vi "Test at 5 second intervals.vi"() -> ()   [LabVIEW 2018]
uses:
  <vilib>/Plasmionique/MB Master/MB_Master_TCP/MB_Master_TCP.lvclass
  C:/Program Files (x86)/National Instruments/LabVIEW 2018/vi.lib/Plasmionique/MB Master/MB_Master/MB_Master.lvclass
  <vilib>/Plasmionique/MB Master/MB Master.lvlib
panel:
  in  "Delay Curtailment and Power Factor":bool
  in  "Stop Button":bool
  out "Done":bool
  in  "No Delay Curtailment and Power Factor":bool
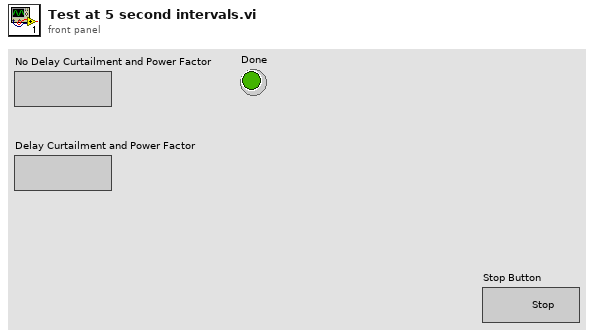
[diagram p1: front panel]
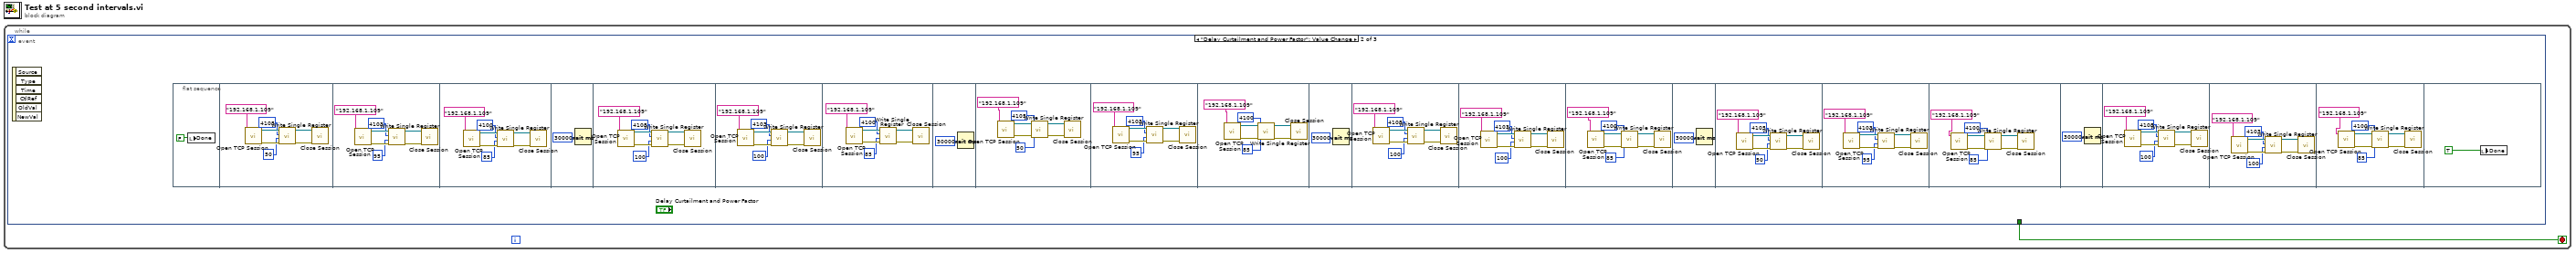
[diagram p0: block diagram]
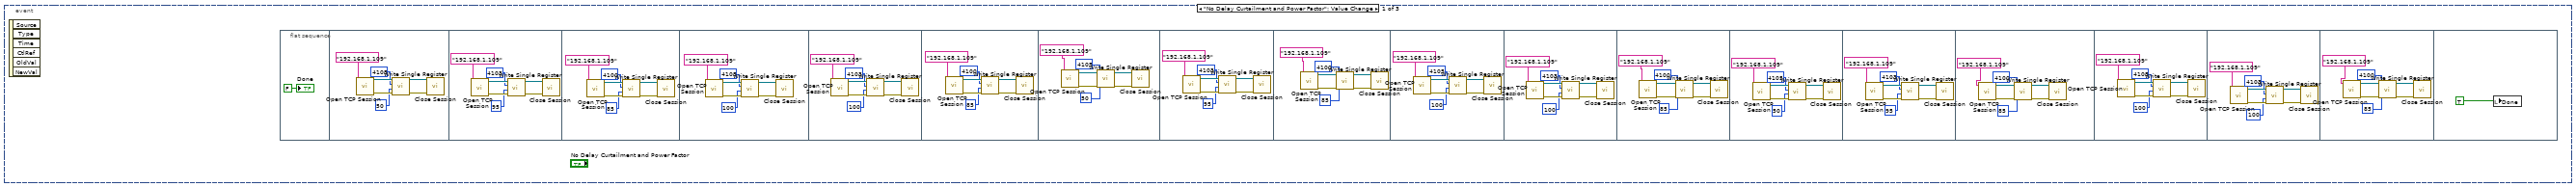
[diagram p2: hidden frame]
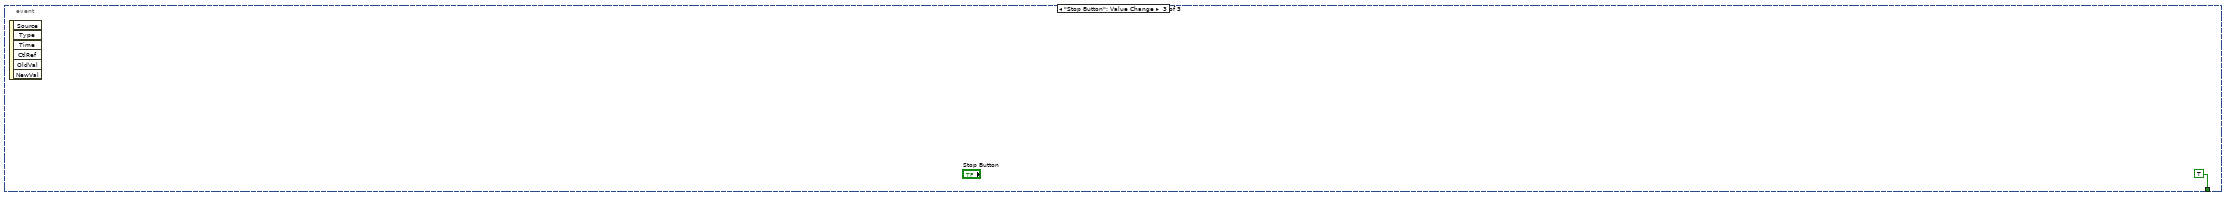
[diagram p3: hidden frame]
diagram:
  n1 = while {
    stop <- w1 stop-if-true
    n2 = event shown="[1] \"Delay Curtailment and Power Factor\": Value Change" {
      selector: _ -> [_ _ _]
      dyn-events: _ -> [_ _ _]
      timeout: _ -> [_ _ _]
      tunnel: [_ _ TRUE] -> w1
      event "No Delay Curtailment and Power Factor": Value Change {
        n3 = event-data() -> ()  [unwired: 1 in, 6 out]
        n4 = flat-sequence {
          frame #0 {
            "Done" <- FALSE ("Done")
          }
          frame #1 {
            n5 = call <vilib>:"Open TCP Session.vi"("IP Address"="192.168.1.109") -> ("error out"=w7:errorcluster, "MB_TCP session"=w9:refnum<class "MB_Master_TCP.lvclass">)  [unwired: 9 in]
            n6 = call <vilib>:"Write Single Register.vi"("error in (no error)"=w7, "value"=u16 50, "address"=u16 4105, "MB session in"=w9) -> ("error out"=w6:errorcluster, "MB session out"=w8:refnum<class "MB_Master_TCP.lvclass">)  [unwired: 6 in]
            n7 = call-dynamic "Close Session.vi"("error in (no error)"=w6, "MB TCP session"=w8) -> ()  [unwired: 9 in, 1 out]
          }
          frame #2 {
            n8 = call <vilib>:"Open TCP Session.vi"("IP Address"="192.168.1.109") -> ("error out"=w14:errorcluster, "MB_TCP session"=w16:refnum<class "MB_Master_TCP.lvclass">)  [unwired: 9 in]
            n9 = call <vilib>:"Write Single Register.vi"("error in (no error)"=w14, "value"=u16 95, "address"=u16 4103, "MB session in"=w16) -> ("error out"=w13:errorcluster, "MB session out"=w15:refnum<class "MB_Master_TCP.lvclass">)  [unwired: 6 in]
            n10 = call-dynamic "Close Session.vi"("error in (no error)"=w13, "MB TCP session"=w15) -> ()  [unwired: 9 in, 1 out]
          }
          frame #3 {
            n11 = call <vilib>:"Open TCP Session.vi"("IP Address"="192.168.1.109") -> ("error out"=w21:errorcluster, "MB_TCP session"=w23:refnum<class "MB_Master_TCP.lvclass">)  [unwired: 9 in]
            n12 = call <vilib>:"Write Single Register.vi"("error in (no error)"=w21, "value"=u16 85, "address"=u16 4100, "MB session in"=w23) -> ("error out"=w20:errorcluster, "MB session out"=w22:refnum<class "MB_Master_TCP.lvclass">)  [unwired: 6 in]
            n13 = call-dynamic "Close Session.vi"("error in (no error)"=w20, "MB TCP session"=w22) -> ()  [unwired: 9 in, 1 out]
          }
          frame #4 {
            n14 = call <vilib>:"Open TCP Session.vi"("IP Address"="192.168.1.109") -> ("error out"=w28:errorcluster, "MB_TCP session"=w30:refnum<class "MB_Master_TCP.lvclass">)  [unwired: 9 in]
            n15 = call <vilib>:"Write Single Register.vi"("error in (no error)"=w28, "value"=u16 100, "address"=u16 4105, "MB session in"=w30) -> ("error out"=w27:errorcluster, "MB session out"=w29:refnum<class "MB_Master_TCP.lvclass">)  [unwired: 6 in]
            n16 = call-dynamic "Close Session.vi"("error in (no error)"=w27, "MB TCP session"=w29) -> ()  [unwired: 9 in, 1 out]
          }
          frame #5 {
            n17 = call <vilib>:"Open TCP Session.vi"("IP Address"="192.168.1.109") -> ("error out"=w35:errorcluster, "MB_TCP session"=w37:refnum<class "MB_Master_TCP.lvclass">)  [unwired: 9 in]
            n18 = call <vilib>:"Write Single Register.vi"("error in (no error)"=w35, "value"=u16 100, "address"=u16 4103, "MB session in"=w37) -> ("error out"=w34:errorcluster, "MB session out"=w36:refnum<class "MB_Master_TCP.lvclass">)  [unwired: 6 in]
            n19 = call-dynamic "Close Session.vi"("error in (no error)"=w34, "MB TCP session"=w36) -> ()  [unwired: 9 in, 1 out]
          }
          frame #6 {
            n20 = call <vilib>:"Open TCP Session.vi"("IP Address"="192.168.1.109") -> ("error out"=w42:errorcluster, "MB_TCP session"=w44:refnum<class "MB_Master_TCP.lvclass">)  [unwired: 9 in]
            n21 = call <vilib>:"Write Single Register.vi"("error in (no error)"=w42, "value"=u16 85, "address"=u16 4100, "MB session in"=w44) -> ("error out"=w41:errorcluster, "MB session out"=w43:refnum<class "MB_Master_TCP.lvclass">)  [unwired: 6 in]
            n22 = call-dynamic "Close Session.vi"("error in (no error)"=w41, "MB TCP session"=w43) -> ()  [unwired: 9 in, 1 out]
          }
          frame #7 {
            n23 = call <vilib>:"Open TCP Session.vi"("IP Address"="192.168.1.109") -> ("error out"=w50:errorcluster, "MB_TCP session"=w48:refnum<class "MB_Master_TCP.lvclass">)  [unwired: 9 in]
            n24 = call <vilib>:"Write Single Register.vi"("error in (no error)"=w50, "value"=u16 50, "address"=u16 4105, "MB session in"=w48) -> ("error out"=w51:errorcluster, "MB session out"=w49:refnum<class "MB_Master_TCP.lvclass">)  [unwired: 6 in]
            n25 = call-dynamic "Close Session.vi"("error in (no error)"=w51, "MB TCP session"=w49) -> ()  [unwired: 9 in, 1 out]
          }
          frame #8 {
            n26 = call <vilib>:"Open TCP Session.vi"("IP Address"="192.168.1.109") -> ("error out"=w56:errorcluster, "MB_TCP session"=w58:refnum<class "MB_Master_TCP.lvclass">)  [unwired: 9 in]
            n27 = call <vilib>:"Write Single Register.vi"("error in (no error)"=w56, "value"=u16 95, "address"=u16 4103, "MB session in"=w58) -> ("error out"=w55:errorcluster, "MB session out"=w57:refnum<class "MB_Master_TCP.lvclass">)  [unwired: 6 in]
            n28 = call-dynamic "Close Session.vi"("error in (no error)"=w55, "MB TCP session"=w57) -> ()  [unwired: 9 in, 1 out]
          }
          frame #9 {
            n29 = call <vilib>:"Open TCP Session.vi"("IP Address"="192.168.1.109") -> ("error out"=w63:errorcluster, "MB_TCP session"=w65:refnum<class "MB_Master_TCP.lvclass">)  [unwired: 9 in]
            n30 = call <vilib>:"Write Single Register.vi"("error in (no error)"=w63, "value"=u16 85, "address"=u16 4100, "MB session in"=w65) -> ("error out"=w62:errorcluster, "MB session out"=w64:refnum<class "MB_Master_TCP.lvclass">)  [unwired: 6 in]
            n31 = call-dynamic "Close Session.vi"("error in (no error)"=w62, "MB TCP session"=w64) -> ()  [unwired: 9 in, 1 out]
          }
          frame #10 {
            n32 = call <vilib>:"Open TCP Session.vi"("IP Address"="192.168.1.109") -> ("error out"=w70:errorcluster, "MB_TCP session"=w72:refnum<class "MB_Master_TCP.lvclass">)  [unwired: 9 in]
            n33 = call <vilib>:"Write Single Register.vi"("error in (no error)"=w70, "value"=u16 100, "address"=u16 4105, "MB session in"=w72) -> ("error out"=w69:errorcluster, "MB session out"=w71:refnum<class "MB_Master_TCP.lvclass">)  [unwired: 6 in]
            n34 = call-dynamic "Close Session.vi"("error in (no error)"=w69, "MB TCP session"=w71) -> ()  [unwired: 9 in, 1 out]
          }
          frame #11 {
            n35 = call <vilib>:"Open TCP Session.vi"("IP Address"="192.168.1.109") -> ("error out"=w77:errorcluster, "MB_TCP session"=w79:refnum<class "MB_Master_TCP.lvclass">)  [unwired: 9 in]
            n36 = call <vilib>:"Write Single Register.vi"("error in (no error)"=w77, "value"=u16 100, "address"=u16 4103, "MB session in"=w79) -> ("error out"=w76:errorcluster, "MB session out"=w78:refnum<class "MB_Master_TCP.lvclass">)  [unwired: 6 in]
            n37 = call-dynamic "Close Session.vi"("error in (no error)"=w76, "MB TCP session"=w78) -> ()  [unwired: 9 in, 1 out]
          }
          frame #12 {
            n38 = call <vilib>:"Open TCP Session.vi"("IP Address"="192.168.1.109") -> ("error out"=w84:errorcluster, "MB_TCP session"=w86:refnum<class "MB_Master_TCP.lvclass">)  [unwired: 9 in]
            n39 = call <vilib>:"Write Single Register.vi"("error in (no error)"=w84, "value"=u16 85, "address"=u16 4100, "MB session in"=w86) -> ("error out"=w83:errorcluster, "MB session out"=w85:refnum<class "MB_Master_TCP.lvclass">)  [unwired: 6 in]
            n40 = call-dynamic "Close Session.vi"("error in (no error)"=w83, "MB TCP session"=w85) -> ()  [unwired: 9 in, 1 out]
          }
          frame #13 {
            n41 = call <vilib>:"Open TCP Session.vi"("IP Address"="192.168.1.109") -> ("error out"=w91:errorcluster, "MB_TCP session"=w93:refnum<class "MB_Master_TCP.lvclass">)  [unwired: 9 in]
            n42 = call <vilib>:"Write Single Register.vi"("error in (no error)"=w91, "value"=u16 50, "address"=u16 4105, "MB session in"=w93) -> ("error out"=w90:errorcluster, "MB session out"=w92:refnum<class "MB_Master_TCP.lvclass">)  [unwired: 6 in]
            n43 = call-dynamic "Close Session.vi"("error in (no error)"=w90, "MB TCP session"=w92) -> ()  [unwired: 9 in, 1 out]
          }
          frame #14 {
            n44 = call <vilib>:"Open TCP Session.vi"("IP Address"="192.168.1.109") -> ("error out"=w98:errorcluster, "MB_TCP session"=w100:refnum<class "MB_Master_TCP.lvclass">)  [unwired: 9 in]
            n45 = call <vilib>:"Write Single Register.vi"("error in (no error)"=w98, "value"=u16 95, "address"=u16 4103, "MB session in"=w100) -> ("error out"=w97:errorcluster, "MB session out"=w99:refnum<class "MB_Master_TCP.lvclass">)  [unwired: 6 in]
            n46 = call-dynamic "Close Session.vi"("error in (no error)"=w97, "MB TCP session"=w99) -> ()  [unwired: 9 in, 1 out]
          }
          frame #15 {
            n47 = call <vilib>:"Open TCP Session.vi"("IP Address"="192.168.1.109") -> ("error out"=w105:errorcluster, "MB_TCP session"=w107:refnum<class "MB_Master_TCP.lvclass">)  [unwired: 9 in]
            n48 = call <vilib>:"Write Single Register.vi"("error in (no error)"=w105, "value"=u16 85, "address"=u16 4100, "MB session in"=w107) -> ("error out"=w104:errorcluster, "MB session out"=w106:refnum<class "MB_Master_TCP.lvclass">)  [unwired: 6 in]
            n49 = call-dynamic "Close Session.vi"("error in (no error)"=w104, "MB TCP session"=w106) -> ()  [unwired: 9 in, 1 out]
          }
          frame #16 {
            n50 = call <vilib>:"Open TCP Session.vi"("IP Address"="192.168.1.109") -> ("error out"=w112:errorcluster, "MB_TCP session"=w114:refnum<class "MB_Master_TCP.lvclass">)  [unwired: 9 in]
            n51 = call <vilib>:"Write Single Register.vi"("error in (no error)"=w112, "value"=u16 100, "address"=u16 4105, "MB session in"=w114) -> ("error out"=w111:errorcluster, "MB session out"=w113:refnum<class "MB_Master_TCP.lvclass">)  [unwired: 6 in]
            n52 = call-dynamic "Close Session.vi"("error in (no error)"=w111, "MB TCP session"=w113) -> ()  [unwired: 9 in, 1 out]
          }
          frame #17 {
            n53 = call <vilib>:"Open TCP Session.vi"("IP Address"="192.168.1.109") -> ("error out"=w119:errorcluster, "MB_TCP session"=w121:refnum<class "MB_Master_TCP.lvclass">)  [unwired: 9 in]
            n54 = call <vilib>:"Write Single Register.vi"("error in (no error)"=w119, "value"=u16 100, "address"=u16 4103, "MB session in"=w121) -> ("error out"=w118:errorcluster, "MB session out"=w120:refnum<class "MB_Master_TCP.lvclass">)  [unwired: 6 in]
            n55 = call-dynamic "Close Session.vi"("error in (no error)"=w118, "MB TCP session"=w120) -> ()  [unwired: 9 in, 1 out]
          }
          frame #18 {
            n56 = call <vilib>:"Open TCP Session.vi"("IP Address"="192.168.1.109") -> ("error out"=w126:errorcluster, "MB_TCP session"=w128:refnum<class "MB_Master_TCP.lvclass">)  [unwired: 9 in]
            n57 = call <vilib>:"Write Single Register.vi"("error in (no error)"=w126, "value"=u16 85, "address"=u16 4100, "MB session in"=w128) -> ("error out"=w125:errorcluster, "MB session out"=w127:refnum<class "MB_Master_TCP.lvclass">)  [unwired: 6 in]
            n58 = call-dynamic "Close Session.vi"("error in (no error)"=w125, "MB TCP session"=w127) -> ()  [unwired: 9 in, 1 out]
          }
          frame #19 {
            n59 = local write "Done"(TRUE ("No Delay Curtailment")) -> ()
          }
        }
      }
      event "Delay Curtailment and Power Factor": Value Change {
        n60 = event-data() -> ()  [unwired: 1 in, 6 out]
        n61 = flat-sequence {
          frame #0 {
            n62 = local write "Done"(FALSE ("Done")) -> ()
          }
          frame #1 {
            n63 = call <vilib>:"Open TCP Session.vi"("IP Address"="192.168.1.109") -> ("error out"=w135:errorcluster, "MB_TCP session"=w137:refnum<class "MB_Master_TCP.lvclass">)  [unwired: 9 in]
            n64 = call <vilib>:"Write Single Register.vi"("error in (no error)"=w135, "value"=u16 50, "address"=u16 4105, "MB session in"=w137) -> ("error out"=w134:errorcluster, "MB session out"=w136:refnum<class "MB_Master_TCP.lvclass">)  [unwired: 6 in]
            n65 = call-dynamic "Close Session.vi"("error in (no error)"=w134, "MB TCP session"=w136) -> ()  [unwired: 9 in, 1 out]
          }
          frame #2 {
            n66 = call <vilib>:"Open TCP Session.vi"("IP Address"="192.168.1.109") -> ("error out"=w142:errorcluster, "MB_TCP session"=w144:refnum<class "MB_Master_TCP.lvclass">)  [unwired: 9 in]
            n67 = call <vilib>:"Write Single Register.vi"("error in (no error)"=w142, "value"=u16 95, "address"=u16 4103, "MB session in"=w144) -> ("error out"=w141:errorcluster, "MB session out"=w143:refnum<class "MB_Master_TCP.lvclass">)  [unwired: 6 in]
            n68 = call-dynamic "Close Session.vi"("error in (no error)"=w141, "MB TCP session"=w143) -> ()  [unwired: 9 in, 1 out]
          }
          frame #3 {
            n69 = call <vilib>:"Open TCP Session.vi"("IP Address"="192.168.1.109") -> ("error out"=w149:errorcluster, "MB_TCP session"=w151:refnum<class "MB_Master_TCP.lvclass">)  [unwired: 9 in]
            n70 = call <vilib>:"Write Single Register.vi"("error in (no error)"=w149, "value"=u16 85, "address"=u16 4100, "MB session in"=w151) -> ("error out"=w148:errorcluster, "MB session out"=w150:refnum<class "MB_Master_TCP.lvclass">)  [unwired: 6 in]
            n71 = call-dynamic "Close Session.vi"("error in (no error)"=w148, "MB TCP session"=w150) -> ()  [unwired: 9 in, 1 out]
          }
          frame #4 {
            n72 = Wait (ms)(milliseconds to wait=u32 30000 ("millisecond timer value")) -> ()  [unwired: 1 out]
          }
          frame #5 {
            n73 = call <vilib>:"Open TCP Session.vi"("IP Address"="192.168.1.109") -> ("error out"=w157:errorcluster, "MB_TCP session"=w159:refnum<class "MB_Master_TCP.lvclass">)  [unwired: 9 in]
            n74 = call <vilib>:"Write Single Register.vi"("error in (no error)"=w157, "value"=u16 100, "address"=u16 4105, "MB session in"=w159) -> ("error out"=w156:errorcluster, "MB session out"=w158:refnum<class "MB_Master_TCP.lvclass">)  [unwired: 6 in]
            n75 = call-dynamic "Close Session.vi"("error in (no error)"=w156, "MB TCP session"=w158) -> ()  [unwired: 9 in, 1 out]
          }
          frame #6 {
            n76 = call <vilib>:"Open TCP Session.vi"("IP Address"="192.168.1.109") -> ("error out"=w164:errorcluster, "MB_TCP session"=w166:refnum<class "MB_Master_TCP.lvclass">)  [unwired: 9 in]
            n77 = call <vilib>:"Write Single Register.vi"("error in (no error)"=w164, "value"=u16 100, "address"=u16 4103, "MB session in"=w166) -> ("error out"=w163:errorcluster, "MB session out"=w165:refnum<class "MB_Master_TCP.lvclass">)  [unwired: 6 in]
            n78 = call-dynamic "Close Session.vi"("error in (no error)"=w163, "MB TCP session"=w165) -> ()  [unwired: 9 in, 1 out]
          }
          frame #7 {
            n79 = call <vilib>:"Open TCP Session.vi"("IP Address"="192.168.1.109") -> ("error out"=w171:errorcluster, "MB_TCP session"=w173:refnum<class "MB_Master_TCP.lvclass">)  [unwired: 9 in]
            n80 = call <vilib>:"Write Single Register.vi"("error in (no error)"=w171, "value"=u16 85, "address"=u16 4100, "MB session in"=w173) -> ("error out"=w170:errorcluster, "MB session out"=w172:refnum<class "MB_Master_TCP.lvclass">)  [unwired: 6 in]
            n81 = call-dynamic "Close Session.vi"("error in (no error)"=w170, "MB TCP session"=w172) -> ()  [unwired: 9 in, 1 out]
          }
          frame #8 {
            n82 = Wait (ms)(milliseconds to wait=u32 30000 ("millisecond timer value")) -> ()  [unwired: 1 out]
          }
          frame #9 {
            n83 = call <vilib>:"Open TCP Session.vi"("IP Address"="192.168.1.109") -> ("error out"=w180:errorcluster, "MB_TCP session"=w178:refnum<class "MB_Master_TCP.lvclass">)  [unwired: 9 in]
            n84 = call <vilib>:"Write Single Register.vi"("error in (no error)"=w180, "value"=u16 50, "address"=u16 4105, "MB session in"=w178) -> ("error out"=w181:errorcluster, "MB session out"=w179:refnum<class "MB_Master_TCP.lvclass">)  [unwired: 6 in]
            n85 = call-dynamic "Close Session.vi"("error in (no error)"=w181, "MB TCP session"=w179) -> ()  [unwired: 9 in, 1 out]
          }
          frame #10 {
            n86 = call <vilib>:"Open TCP Session.vi"("IP Address"="192.168.1.109") -> ("error out"=w186:errorcluster, "MB_TCP session"=w188:refnum<class "MB_Master_TCP.lvclass">)  [unwired: 9 in]
            n87 = call <vilib>:"Write Single Register.vi"("error in (no error)"=w186, "value"=u16 95, "address"=u16 4103, "MB session in"=w188) -> ("error out"=w185:errorcluster, "MB session out"=w187:refnum<class "MB_Master_TCP.lvclass">)  [unwired: 6 in]
            n88 = call-dynamic "Close Session.vi"("error in (no error)"=w185, "MB TCP session"=w187) -> ()  [unwired: 9 in, 1 out]
          }
          frame #11 {
            n89 = call <vilib>:"Open TCP Session.vi"("IP Address"="192.168.1.109") -> ("error out"=w193:errorcluster, "MB_TCP session"=w195:refnum<class "MB_Master_TCP.lvclass">)  [unwired: 9 in]
            n90 = call <vilib>:"Write Single Register.vi"("error in (no error)"=w193, "value"=u16 85, "address"=u16 4100, "MB session in"=w195) -> ("error out"=w192:errorcluster, "MB session out"=w194:refnum<class "MB_Master_TCP.lvclass">)  [unwired: 6 in]
            n91 = call-dynamic "Close Session.vi"("error in (no error)"=w192, "MB TCP session"=w194) -> ()  [unwired: 9 in, 1 out]
          }
          frame #12 {
            n92 = Wait (ms)(milliseconds to wait=u32 30000 ("millisecond timer value")) -> ()  [unwired: 1 out]
          }
          frame #13 {
            n93 = call <vilib>:"Open TCP Session.vi"("IP Address"="192.168.1.109") -> ("error out"=w201:errorcluster, "MB_TCP session"=w203:refnum<class "MB_Master_TCP.lvclass">)  [unwired: 9 in]
            n94 = call <vilib>:"Write Single Register.vi"("error in (no error)"=w201, "value"=u16 100, "address"=u16 4105, "MB session in"=w203) -> ("error out"=w200:errorcluster, "MB session out"=w202:refnum<class "MB_Master_TCP.lvclass">)  [unwired: 6 in]
            n95 = call-dynamic "Close Session.vi"("error in (no error)"=w200, "MB TCP session"=w202) -> ()  [unwired: 9 in, 1 out]
          }
          frame #14 {
            n96 = call <vilib>:"Open TCP Session.vi"("IP Address"="192.168.1.109") -> ("error out"=w208:errorcluster, "MB_TCP session"=w210:refnum<class "MB_Master_TCP.lvclass">)  [unwired: 9 in]
            n97 = call <vilib>:"Write Single Register.vi"("error in (no error)"=w208, "value"=u16 100, "address"=u16 4103, "MB session in"=w210) -> ("error out"=w207:errorcluster, "MB session out"=w209:refnum<class "MB_Master_TCP.lvclass">)  [unwired: 6 in]
            n98 = call-dynamic "Close Session.vi"("error in (no error)"=w207, "MB TCP session"=w209) -> ()  [unwired: 9 in, 1 out]
          }
          frame #15 {
            n99 = call <vilib>:"Open TCP Session.vi"("IP Address"="192.168.1.109") -> ("error out"=w215:errorcluster, "MB_TCP session"=w217:refnum<class "MB_Master_TCP.lvclass">)  [unwired: 9 in]
            n100 = call <vilib>:"Write Single Register.vi"("error in (no error)"=w215, "value"=u16 85, "address"=u16 4100, "MB session in"=w217) -> ("error out"=w214:errorcluster, "MB session out"=w216:refnum<class "MB_Master_TCP.lvclass">)  [unwired: 6 in]
            n101 = call-dynamic "Close Session.vi"("error in (no error)"=w214, "MB TCP session"=w216) -> ()  [unwired: 9 in, 1 out]
          }
          frame #16 {
            n102 = Wait (ms)(milliseconds to wait=u32 30000 ("millisecond timer value")) -> ()  [unwired: 1 out]
          }
          frame #17 {
            n103 = call <vilib>:"Open TCP Session.vi"("IP Address"="192.168.1.109") -> ("error out"=w223:errorcluster, "MB_TCP session"=w225:refnum<class "MB_Master_TCP.lvclass">)  [unwired: 9 in]
            n104 = call <vilib>:"Write Single Register.vi"("error in (no error)"=w223, "value"=u16 50, "address"=u16 4105, "MB session in"=w225) -> ("error out"=w222:errorcluster, "MB session out"=w224:refnum<class "MB_Master_TCP.lvclass">)  [unwired: 6 in]
            n105 = call-dynamic "Close Session.vi"("error in (no error)"=w222, "MB TCP session"=w224) -> ()  [unwired: 9 in, 1 out]
          }
          frame #18 {
            n106 = call <vilib>:"Open TCP Session.vi"("IP Address"="192.168.1.109") -> ("error out"=w230:errorcluster, "MB_TCP session"=w232:refnum<class "MB_Master_TCP.lvclass">)  [unwired: 9 in]
            n107 = call <vilib>:"Write Single Register.vi"("error in (no error)"=w230, "value"=u16 95, "address"=u16 4103, "MB session in"=w232) -> ("error out"=w229:errorcluster, "MB session out"=w231:refnum<class "MB_Master_TCP.lvclass">)  [unwired: 6 in]
            n108 = call-dynamic "Close Session.vi"("error in (no error)"=w229, "MB TCP session"=w231) -> ()  [unwired: 9 in, 1 out]
          }
          frame #19 {
            n109 = call <vilib>:"Open TCP Session.vi"("IP Address"="192.168.1.109") -> ("error out"=w237:errorcluster, "MB_TCP session"=w239:refnum<class "MB_Master_TCP.lvclass">)  [unwired: 9 in]
            n110 = call <vilib>:"Write Single Register.vi"("error in (no error)"=w237, "value"=u16 85, "address"=u16 4100, "MB session in"=w239) -> ("error out"=w236:errorcluster, "MB session out"=w238:refnum<class "MB_Master_TCP.lvclass">)  [unwired: 6 in]
            n111 = call-dynamic "Close Session.vi"("error in (no error)"=w236, "MB TCP session"=w238) -> ()  [unwired: 9 in, 1 out]
          }
          frame #20 {
            n112 = Wait (ms)(milliseconds to wait=u32 30000 ("millisecond timer value")) -> ()  [unwired: 1 out]
          }
          frame #21 {
            n113 = call <vilib>:"Open TCP Session.vi"("IP Address"="192.168.1.109") -> ("error out"=w245:errorcluster, "MB_TCP session"=w247:refnum<class "MB_Master_TCP.lvclass">)  [unwired: 9 in]
            n114 = call <vilib>:"Write Single Register.vi"("error in (no error)"=w245, "value"=u16 100, "address"=u16 4105, "MB session in"=w247) -> ("error out"=w244:errorcluster, "MB session out"=w246:refnum<class "MB_Master_TCP.lvclass">)  [unwired: 6 in]
            n115 = call-dynamic "Close Session.vi"("error in (no error)"=w244, "MB TCP session"=w246) -> ()  [unwired: 9 in, 1 out]
          }
          frame #22 {
            n116 = call <vilib>:"Open TCP Session.vi"("IP Address"="192.168.1.109") -> ("error out"=w252:errorcluster, "MB_TCP session"=w254:refnum<class "MB_Master_TCP.lvclass">)  [unwired: 9 in]
            n117 = call <vilib>:"Write Single Register.vi"("error in (no error)"=w252, "value"=u16 100, "address"=u16 4103, "MB session in"=w254) -> ("error out"=w251:errorcluster, "MB session out"=w253:refnum<class "MB_Master_TCP.lvclass">)  [unwired: 6 in]
            n118 = call-dynamic "Close Session.vi"("error in (no error)"=w251, "MB TCP session"=w253) -> ()  [unwired: 9 in, 1 out]
          }
          frame #23 {
            n119 = call <vilib>:"Open TCP Session.vi"("IP Address"="192.168.1.109") -> ("error out"=w259:errorcluster, "MB_TCP session"=w261:refnum<class "MB_Master_TCP.lvclass">)  [unwired: 9 in]
            n120 = call <vilib>:"Write Single Register.vi"("error in (no error)"=w259, "value"=u16 85, "address"=u16 4100, "MB session in"=w261) -> ("error out"=w258:errorcluster, "MB session out"=w260:refnum<class "MB_Master_TCP.lvclass">)  [unwired: 6 in]
            n121 = call-dynamic "Close Session.vi"("error in (no error)"=w258, "MB TCP session"=w260) -> ()  [unwired: 9 in, 1 out]
          }
          frame #24 {
            n122 = local write "Done"(TRUE ("No Delay Curtailment")) -> ()
          }
        }
      }
      event "Stop Button": Value Change {
        n123 = event-data() -> ()  [unwired: 1 in, 6 out]
      }
    }
  }
